vi "TDR_setup.vi"(0 "VISA IN":refnum<visa-resource-name>="GPIB0::16::INSTR", 2 "FileName":string="MyFile", 5 "error in":errorcluster, 7 "Channel":i32=1) -> (14 "dup VISA session":refnum<visa-resource-name>="GPIB0::16::INSTR", 15 "StartT":dbl, 16 "StopT":dbl, 17 "Num Pts":dbl=401.0, 19 "error out":errorcluster)   [LabVIEW 2018]
uses:
  PNA-X.lvlib
panel:
  in  "UNIT":string(combo)="INCH"
  in  "MODE":string(combo)="AUTO"
  in  "Window Width(0-13 sec)":dbl=1.0 min=0.0 max=13.0
  in  "Impulse Width(%)":dbl min=0.0 max=1.0 step=0.1
  in  "Time Domain ON/OFF":bool=TRUE
  out "Span\nIn Range?":bool=TRUE
  in  "Time Domain Trace Coupling":bool=TRUE
  in  "COUPLING":T1={"STIMULUS"=TRUE, "STATE"=TRUE, "WINDOW"=TRUE, "MODE"=TRUE, "MARKER"=TRUE}
  in  "Type":string(combo)="BPAS-IMP"
  in  "Span Time(sec)":dbl=2e-08
  in  "Center Time(sec)":dbl=9e-09
  in  "Fliter_OffOn":bool=TRUE
  in  "FilterShape":string(combo)="NORMal"
  in  "FilterType":string(combo)="BPASs"
  in  "GATING":T2={"STIMULUS"=TRUE, "STATE"=TRUE, "SHAPE"=TRUE, "TYPE"=TRUE}
  in  "Points":dbl=401.0
  in  "Stop Frq.":dbl=4010000000.0
  in  "Start Frq.":dbl=10000000.0
  in  "Window":i32=1
  in  "Trace":i32=1
  # "TRANSFORM CONTROLS"
  # "GATING CONTROLS"
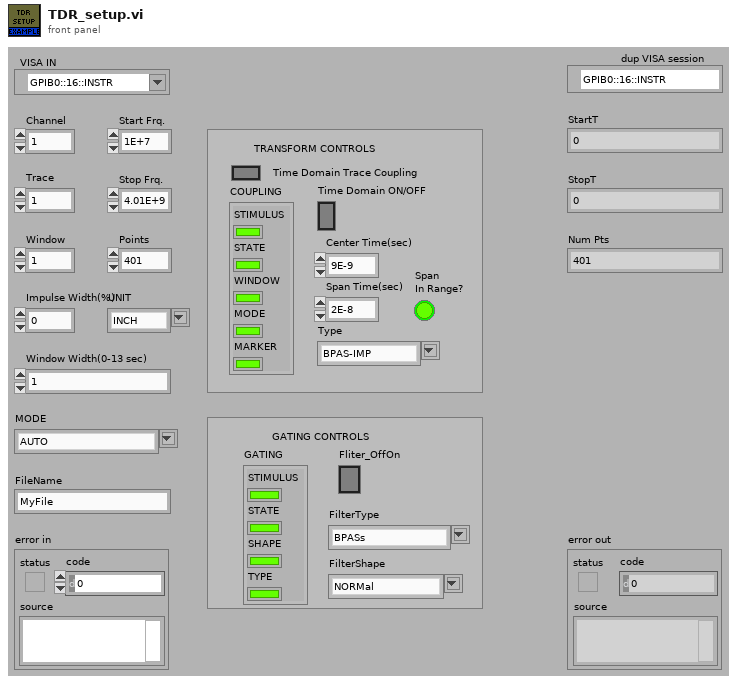
[diagram p1: front panel]
types:
  T1 = cluster{"STIMULUS":bool, "STATE":bool, "WINDOW":bool, "MODE":bool, "MARKER":bool}
  T2 = cluster{"STIMULUS":bool, "STATE":bool, "SHAPE":bool, "TYPE":bool}
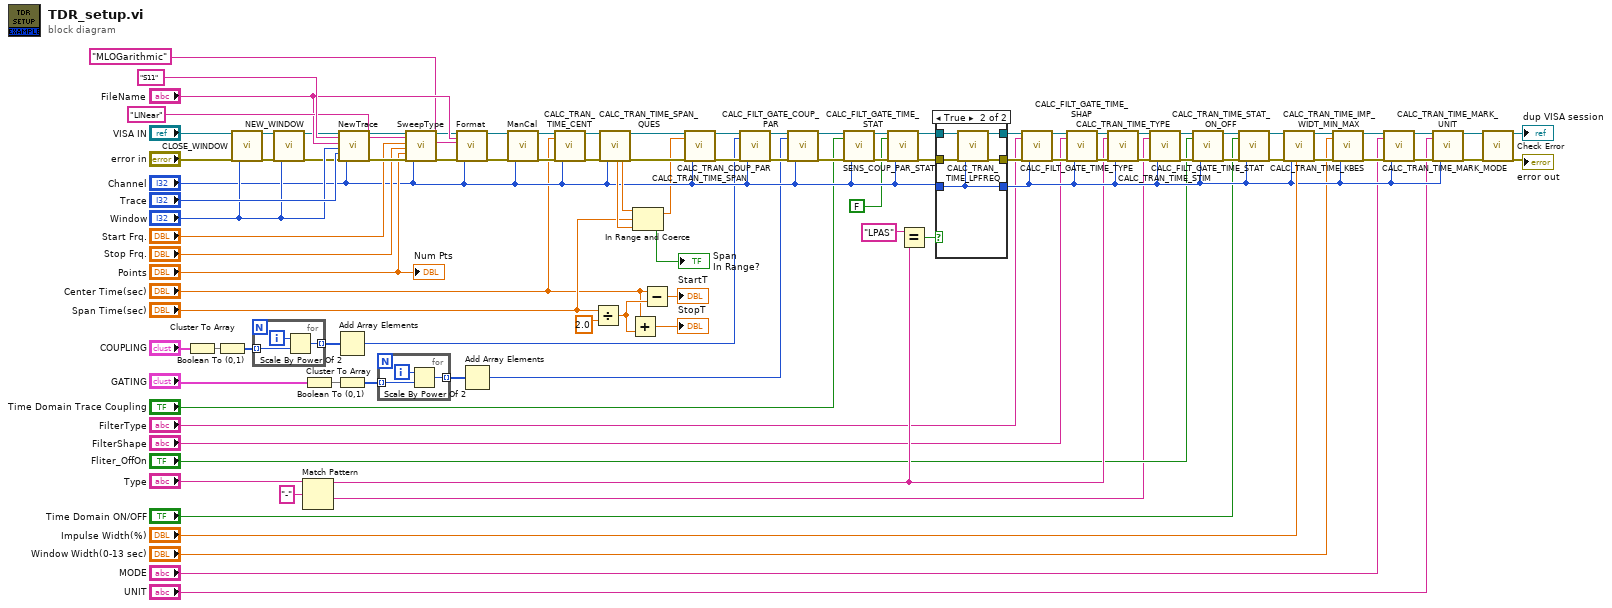
[diagram p0: block diagram]
diagram:
  n1 = Cluster To Array(cluster="COUPLING") -> (array=w75:bool[])
  n2 = Boolean To (0,1)(Boolean=w75) -> (0, 1=w74:i16[])
  n3 = call "CLOSE_WINDOW.vi"("VISA IN"="VISA IN", "error in"="error in", "Window"="Window") -> ("VISA Out"=w85:refnum<visa-resource-name>, "error out"=w87:errorcluster)  [unwired: 15 in]
  n4 = for {
    tunnel: w74 -> [w101] mode=indexing
    tunnel: [w100] -> w73 mode=indexing
    i -> [w102]
    n5 = Scale By Power Of 2(n=w102, x=w101) -> (x*2^n=w100:i16)
  }
  n6 = call "NEW_WINDOW.vi"("VISA IN"=w85, "error in"=w87, "Window"="Window") -> ("VISA Out"=w84:refnum<visa-resource-name>, "error out"=w83:errorcluster)  [unwired: 15 in]
  n7 = Match Pattern(string="Type", regular expression="-") -> (before substring=w10:string, after substring=w1:string)  [unwired: 1 in, 2 out]
  n8 = Cluster To Array(cluster="GATING") -> (array=w68:bool[])
  n9 = Add Array Elements(numeric array=w73) -> (sum=w14:i16)
  n10 = Boolean To (0,1)(Boolean=w68) -> (0, 1=w67:i16[])
  n11 = call "NewTrace.vi"("VISA IN"=w84, "Measurement"="S11", "FileName"="FileName", "Window"="Window", "Trace"="Trace", "error in (no error)"=w83, "Channel"="Channel") -> ("VISA Out"=w94:refnum<visa-resource-name>, "error out"=w95:errorcluster)  [unwired: 11 in]
  n12 = for {
    tunnel: w67 -> [w104] mode=indexing
    tunnel: [w103] -> w66 mode=indexing
    i -> [w105]
    n13 = Scale By Power Of 2(n=w105, x=w104) -> (x*2^n=w103:i16)
  }
  n14 = call "SweepType.vi"("VISA IN"=w94, "Sweep Type"="LINear", "Start Frq."="Start Frq.", "Stop Frq."="Stop Frq.", "Points"="Points", "error in"=w95, "Channel"="Channel") -> ("VISA Out"=w93:refnum<visa-resource-name>, "error out"=w92:errorcluster)  [unwired: 11 in]
  n15 = call "Format.vi"("VISA IN"=w93, "Measurement Name"="FileName", "Format"="MLOGarithmic", "error in"=w92, "Channel"="Channel") -> ("VISA Out"=w29:refnum<visa-resource-name>, "error out"=w27:errorcluster)  [unwired: 13 in]
  n16 = Add Array Elements(numeric array=w66) -> (sum=w13:i16)
  n17 = call "ManCal.vi"("VISA IN"=w29, "error in"=w27, "Channel"="Channel") -> ("VISA Out"=w28:refnum<visa-resource-name>, "error out"=w26:errorcluster)  [unwired: 15 in]
  n18 = call "CALC_TRAN_TIME_CENT.vi"("VISA IN"=w28, "Center Time(sec)"="Center Time(sec)", "error in"=w26, "Channel"="Channel") -> ("VISA Out"=w81:refnum<visa-resource-name>, "error out"=w82:errorcluster)  [unwired: 14 in]
  n19 = Divide(x="Span Time(sec)", y=2.0) -> (x/y=w20:dbl)
  n20 = call "CALC_TRAN_TIME_SPAN_QUES.vi"("VISA IN"=w81, "error in"=w82, "Channel"="Channel") -> ("min"=w78:dbl, "max"=w77:dbl, "VISA Out"=w80:refnum<visa-resource-name>, "error out"=w79:errorcluster)  [unwired: 13 in]
  n21 = Add(x="Center Time(sec)", y=w20) -> (x+y=→"StopT":dbl)
  n22 = In Range and Coerce(upper limit=w77, x="Span Time(sec)", lower limit=w78) -> (coerced(x)=w15:dbl, In Range?=→"Span\nIn Range?":bool)
  n23 = Subtract(x="Center Time(sec)", y=w20) -> (x-y=→"StartT":dbl)
  n24 = call "CALC_TRAN_TIME_SPAN.vi"("VISA IN"=w80, "Span Time(sec)"=w15, "error in"=w79, "Channel"="Channel") -> ("VISA Out"=w71:refnum<visa-resource-name>, "error out"=w72:errorcluster)  [unwired: 14 in]
  n25 = call "CALC_TRAN_COUP_PAR.vi"("VISA IN"=w71, "Parameters to Couple"=w14, "error in"=w72, "Channel"="Channel") -> ("VISA Out"=w69:refnum<visa-resource-name>, "error out"=w70:errorcluster)  [unwired: 14 in]
  n26 = call "CALC_FILT_GATE_COUP_PAR.vi"("VISA IN"=w69, "Parameters"=w13, "error in"=w70, "Channel"="Channel") -> ("VISA Out"=w64:refnum<visa-resource-name>, "error out"=w63:errorcluster)  [unwired: 14 in]
  n27 = call "SENS_COUP_PAR_STAT.vi"("VISA IN"=w64, "Time Domain Trace Coupling ON/OFF"="Time Domain Trace Coupling", "error in"=w63, "Channel"="Channel") -> ("VISA Out"=w56:refnum<visa-resource-name>, "error out"=w55:errorcluster)  [unwired: 14 in]
  n28 = call "CALC_FILT_GATE_TIME_STAT.vi"("VISA IN"=w56, "Cmd 1"=FALSE ("OFF_ON"), "error in"=w55, "Channel"="Channel") -> ("VISA Out"=w51:refnum<visa-resource-name>, "error out"=w53:errorcluster)  [unwired: 14 in]
  n29 = Equal?(x="LPAS", y=w10) -> (x = y?=w49:bool)
  n30 = case shown="True" w49 {
    tunnel: w51 -> [w108 w113]
    tunnel: w53 -> [w107 w112]
    tunnel: "Channel" -> [w106 w109]
    tunnel: [w107 w111] -> w52
    tunnel: [w108 w110] -> w50
    tunnel: [w106 w109] -> w34
    frame False {
    }
    frame True {
      n31 = call "CALC_TRAN_TIME_LPFREQ.vi"("VISA IN"=w113, "error in"=w112, "Channel"=w109) -> ("VISA Out"=w110:refnum<visa-resource-name>, "error out"=w111:errorcluster)  [unwired: 15 in]
    }
  }
  n32 = call "CALC_FILT_GATE_TIME_TYPE.vi"("VISA IN"=w50, "FilterType"="FilterType", "error in"=w52, "Channel"=w34) -> ("VISA Out"=w61:refnum<visa-resource-name>, "error out"=w62:errorcluster)  [unwired: 14 in]
  n33 = call "CALC_FILT_GATE_TIME_SHAP.vi"("VISA IN"=w61, "FilterShape"="FilterShape", "error in"=w62, "Channel"=w34) -> ("VISA Out"=w47:refnum<visa-resource-name>, "error out"=w48:errorcluster)  [unwired: 14 in]
  n34 = call "CALC_TRAN_TIME_TYPE.vi"("VISA IN"=w47, "Type"=w10, "error in"=w48, "Channel"=w34) -> ("VISA Out"=w60:refnum<visa-resource-name>, "error out"=w59:errorcluster)  [unwired: 14 in]
  n35 = call "CALC_TRAN_TIME_STIM.vi"("VISA IN"=w60, "Stimulus"=w1, "error in"=w59, "Channel"=w34) -> ("VISA Out"=w3:refnum<visa-resource-name>, "error out"=w46:errorcluster)  [unwired: 14 in]
  n36 = call "CALC_FILT_GATE_TIME_STAT.vi"("VISA IN"=w3, "Cmd 1"="Fliter_OffOn", "error in"=w46, "Channel"=w34) -> ("VISA Out"=w45:refnum<visa-resource-name>, "error out"=w44:errorcluster)  [unwired: 14 in]
  n37 = call "CALC_TRAN_TIME_STAT_ON_OFF.vi"("VISA IN"=w45, "Time Domain ON/OFF"="Time Domain ON/OFF", "error in"=w44, "Channel"=w34) -> ("VISA Out"=w42:refnum<visa-resource-name>, "error out"=w43:errorcluster)  [unwired: 14 in]
  n38 = call "CALC_TRAN_TIME_IMP_WIDT_MIN_MAX.vi"("VISA IN"=w42, "error in"=w43, "Channel"=w34, "Impulse Width(sec)"="Impulse Width(%)") -> ("VISA Out"=w39:refnum<visa-resource-name>, "error out"=w40:errorcluster)  [unwired: 14 in]
  n39 = call "CALC_TRAN_TIME_KBES.vi"("VISA IN"=w39, "Window Width(sec)"="Window Width(0-13 sec)", "error in"=w40, "Channel"=w34) -> ("VISA Out"=w38:refnum<visa-resource-name>, "error out"=w37:errorcluster)  [unwired: 14 in]
  n40 = call "CALC_TRAN_TIME_MARK_MODE.vi"("VISA IN"=w38, "MODE"="MODE", "error in"=w37, "Channel"=w34) -> ("VISA Out"=w35:refnum<visa-resource-name>, "error out"=w36:errorcluster)  [unwired: 14 in]
  n41 = call "CALC_TRAN_TIME_MARK_UNIT.vi"("VISA IN"=w35, "UNIT"="UNIT", "error in"=w36, "Channel"=w34) -> ("VISA Out"=w33:refnum<visa-resource-name>, "error out"=w32:errorcluster)  [unwired: 14 in]
  n42 = call "Check Error.vi"("VISA Resource Name"=w33, "error in (no error)"=w32) -> ("dup VISA session"=→"dup VISA session":refnum<visa-resource-name>, "error out"=→"error out":errorcluster)  [unwired: 16 in]
  "Num Pts" <- "Points"
